vi "Read Instance.vi"(11 "Dependency in":refnum<class "Dependency.lvclass">) -> (2 "SMO.lvclass":refnum<class "SMO.lvclass">, 3 "Dependency out":refnum<class "Dependency.lvclass">)   [LabVIEW 2019, in "Dependency.lvclass"]
doc: "JKI State Machine Objects (SMO) 1.3.0.56\nJKI - JKI\nCopyright (c) 2017, JKI"
uses:
  Dependency.lvclass
  SMO/SMO.lvclass
  Dependency.lvclass/Dependency.ctl
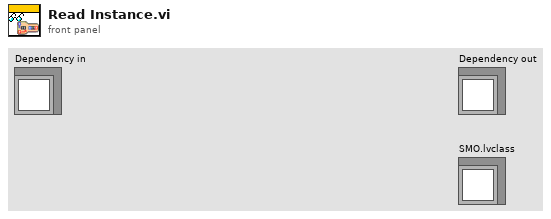
[diagram p1: front panel]
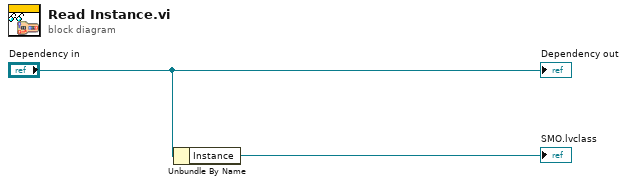
[diagram p0: block diagram]
diagram:
  n1 = Unbundle By Name("Dependency in") -> ("Instance"=→"SMO.lvclass":refnum<class "SMO.lvclass">)
  "Dependency out" <- "Dependency in"
